vi "Queue State & Data.vi"   [LabVIEW 2024, in "ED Queued State Machine.lvlib"]
doc: "This polymorphic VI allows enqueueing states into the state machine queue, either as a single state or as a list of states. In both cases, each state is represented by a string and can optionally be accompanied by an associated data item passed as a Variant.\n\nIn the single-state version, one state is enqueued, by default at the rear of the queue. If priority is required, the state can be enqueued at the front by setting the <b>Priority State? (F)</b> input to True.\n\nIn the array version, a list of states is enqueued, provided as an array of strings. The <b>Priority State Array? (F)</b> input allows specifying, for each individual state, whether it should be inserted at the front or rear of the queue, giving full control over execution order."
uses:
  ED Queued State Machine.lvlib
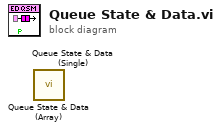
[diagram p0: block diagram]
diagram:
  n1 = call "Queue State & Data (Array).vi"() -> ()  [unwired: 10 in, 2 out]
  n2 = call "Queue State & Data (Single).vi"() -> ()  [unwired: 10 in, 2 out]
